vi "FPGA (Top Level)_torque_control.vi"() -> ()   [LabVIEW 2015]
uses:
  <vilib>/Platform/TimedLoop/XDataNode/wakeup.ctl
  <vilib>/Platform/TimedLoop/XDataNode/XDNodeRunTimeDep.lvlib
  <vilib>/Platform/TimedLoop/XDataNode/nitl_modes.ctl
  <vilib>/Platform/TimedLoop/XDataNode/timing_clust.ctl
  <vilib>/Platform/TimedLoop/XDataNode/XDataNode.xnode
  <vilib>/eio/EIONode/EIONode.xnode
  <vilib>/rvi/eio/common/nirviEmuTemplateMethod_errors.vi
  <vilib>/rvi/DataTransferAndStorage/Container/XNode/niFpgaContainer.xnode
  <vilib>/rvi/DataTransferAndStorage/Register/Emulation/niFpgaRegisterEmulation.vi
  <vilib>/rvi/FXPMathLib/FxpSinAndCos/XNode/nifxpmath_SinAndCos.xnode
  <vilib>/rvi/FXPMathLib/FxpSinAndCos/simVIs/DllFxpSinAndCosTemp_sub.vi
  <vilib>/rvi/FXPMathLib/FxpSinAndCos/subVIs/nifxpmath_SinAndCos_SimConfig.ctl
  <vilib>/eio/EIOMethodNode/EIOMethodNode.xnode
  <vilib>/eio/EIOPropertyNode/EIOPropertyNode.xnode
  <vilib>/rvi/eio/common/nirviEmuTemplatePropertyGet_errors.vi
  <vilib>/rvi/eio/common/nirviEmuTemplatePropertyGet_noerrors.vi
  <vilib>/rvi/eio/common/nirviEmuTemplatePropertySet_errors.vi
  <vilib>/rvi/eio/common/nirviEmuTemplatePropertySet_noerrors.vi
  <vilib>/Motion/MotorControl/_s/nism.pwm.v.dcp.range.fxp.1.15.ctl
  <vilib>/rvi/Analysis/control/PID/SubVIs/niFpgaPID_PIWrapper.vi
  <vilib>/Motion/MotorControl/_s/nism.pwm.center.fxp.vi
  <vilib>/LabVIEW Targets/FPGA/cRIO/cRIO-9505/controls.llb/_nicrio_cRIO-9505_DriveStatus.ctl
  <vilib>/rvi/Analysis/control/PID/Typedef/niFpgaPID_PIGains.ctl
  <vilib>/rvi/Analysis/control/PID/Typedef/niFpgaPID_OutputRange.ctl
panel:
  in  "LINK2_DEMAND_CURRENT":sgl
  out "LINK2_ACTUAL_CURRENT":sgl
  in  "LINK2_PI_GAINS":T1 {"proportional gain" step=0.125}
  in  "LINK2_PI_RANGE":T2={"output high (Inf)"=1.0, "output low (-Inf)"=-1.0}
  in  "LINK1_PI_RANGE":T2={"output high (Inf)"=1.0, "output low (-Inf)"=-1.0}
  in  "LINK1_PI_GAINS":T1 {"proportional gain" step=0.125}
  in  "PWM_FREQ":fxp<+,32,0>
  in  "LINK1_DEMAND_CURRENT":sgl
  out "LINK1_ACTUAL_CURRENT":sgl
  out "LINK2_DRIVE_STATUS":T3
  out "LINK1_DRIVE_STATUS":T3
  in  "LINK2_DRIVE_ENABLED":bool
  in  "LINK1_DRIVE_ENABLED":bool
  in  "LINK2_PID_ENABLED":bool
  in  "LINK1_PID_ENABLED":bool
  in  "LINK2_DEMAND_CURRENT":i16
  in  "LINK1_DEMAND_CURRENT":i16
  out "LINK2_ACTUAL_CURRENT":i16
  out "LINK1_ACTUAL_CURRENT":i16
  out "LINK2_X_MM":fxp<+/-,34,16>
  out "LINK2_Y_MM":fxp<+/-,34,16>
  in  "Y_OFFSET_MM":fxp<+/-,33,15>
  in  "X_OFFSET_MM":fxp<+/-,33,15>
  in  "LINK2_LENGTH_MM":fxp<+,16,12>=2.0 format="%#_19g"
  in  "LINK1_LENGTH_MM":fxp<+,16,12>=2.0 format="%#_19g"
  out "LINK2_POT_POS":i32
  out "LINK1_POT_POS":i32
  out "LINK2_ENC_POS":i32
  out "LINK1_ENC_POS":i32
  in  "LINK2_ENC_SCALE":fxp<+,32,0>=0.029296900611370802 format="%#_32g"
  in  "LINK1_ENC_SCALE":fxp<+,32,0> format="%#_32g"
  in  "LINK2_POT_SCALE":fxp<+/-,32,16>
  in  "LINK2_OFFSET":fxp<+/-,16,16>
  in  "LINK1_OFFSET":fxp<+/-,16,16>
  in  "LINK1_POT_SCALE":fxp<+/-,32,16>
  in  "AI_POT_LOOP_US":u16
  in  "ENC_DEBOUNCE_CYCLES":u16=5
  in  "LINK1_ENC_CNTS":i32
  in  "LINK2_ENC_CNTS":i32
  in  "LINK1_UPDATE_ENC":bool
  in  "LINK2_UPDATE_ENC":bool
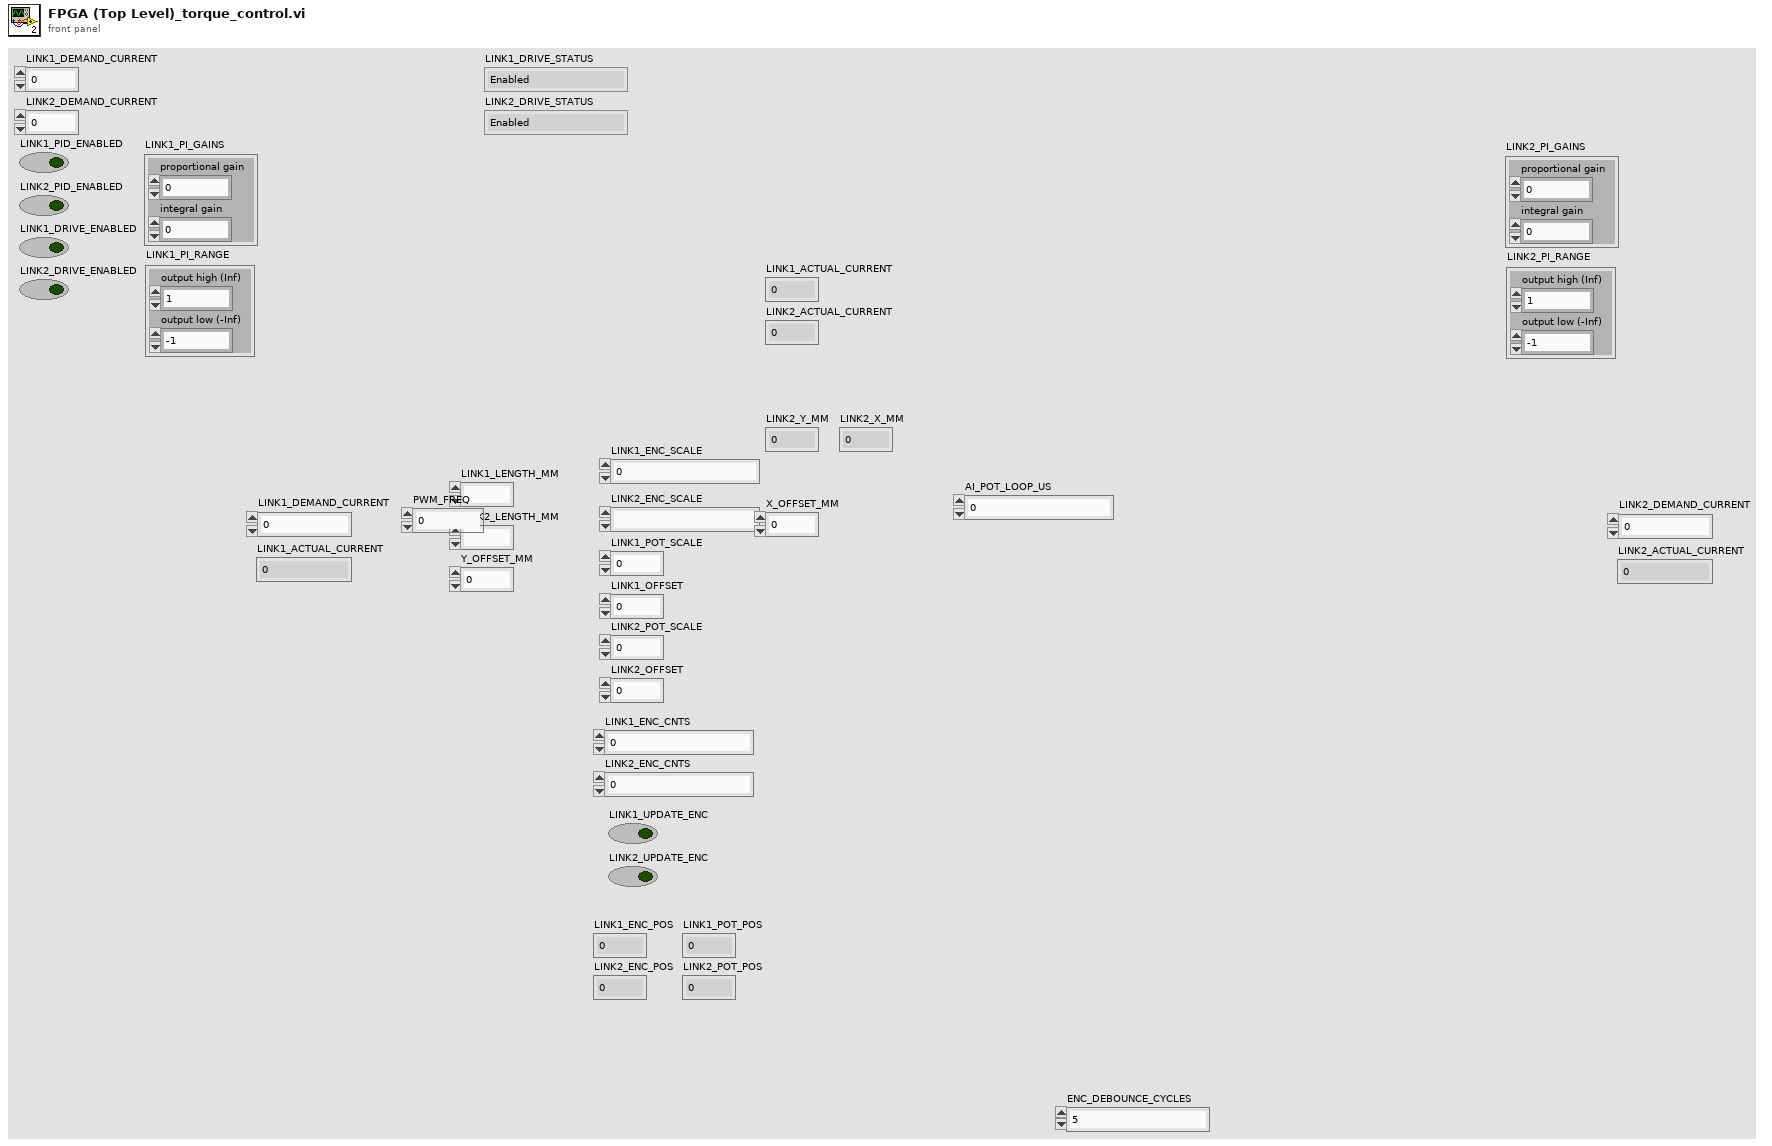
[diagram p1: front panel]
types:
  T1 = typedef "niFpgaPID_PIGains.ctl" = cluster{"proportional gain":sgl, "integral gain":sgl}
  T2 = typedef "niFpgaPID_OutputRange.ctl" = cluster{"output high (Inf)":sgl, "output low (-Inf)":sgl}
  T3 = typedef "_nicrio_cRIO-9505_DriveStatus.ctl" = enum8{"Enabled", "Disabled", "Disabled by Drive Fault", "Disabled by Temp. Fault", "Disabled by E-Stop", "Unknown"}
  T4 = typedef "XDNodeRunTimeDep.lvlib/timing_clust.ctl" = cluster{"Expected End [f-1]":u64, "Actual End [f-1]":u64, "Finished Late? [f-1]":bool, "Expected End [i-1]":u64, "Actual End [i-1]":u64, "Finished Late? [i-1]":bool, "Expected Start [i]":u64, "Actual Start [i]":u64, "Expected Start [f]":u64, "Actual Start [f]":u64, "Source Name":string, "Structure Name":string, "Period":i64, "Deadline":i64, "Offset":i64, "Start":i64, "Priority":i32, "Timeout":i32, "Mode":T5, "Wakeup Reason":T6, "Error":errorcluster, "Source Type":string, "Secondary Source Type":string, "Global End Time":u64, "Global Start Time":u64, "Frame Duration":u64, "Iteration Duration":u64, "Assigned CPU":i32, "I/O Scan Engine Mode":u32}
  T5 = typedef "XDNodeRunTimeDep.lvlib/nitl_modes.ctl" = enum32{"No Change", "Process missed periods, maintain original phase", "Discard missed periods, maintain original phase", "Process missed periods, ignore original phase", "Discard missed periods, ignore original phase"}
  T6 = typedef "XDNodeRunTimeDep.lvlib/wakeup.ctl" = enum32{"Normal", "Aborted", "Asynchronous wakeup", "Timing source error", "Timed loop error", "Timeout"}
  T7 = typedef "NI_SoftMotion_MotorControlIP.lvlib/nism.pwm.v.dcp.range.fxp.1.15.ctl" = cluster{"upper limit":fxp<+,16,1>, "lower limit":fxp<+,16,1>}
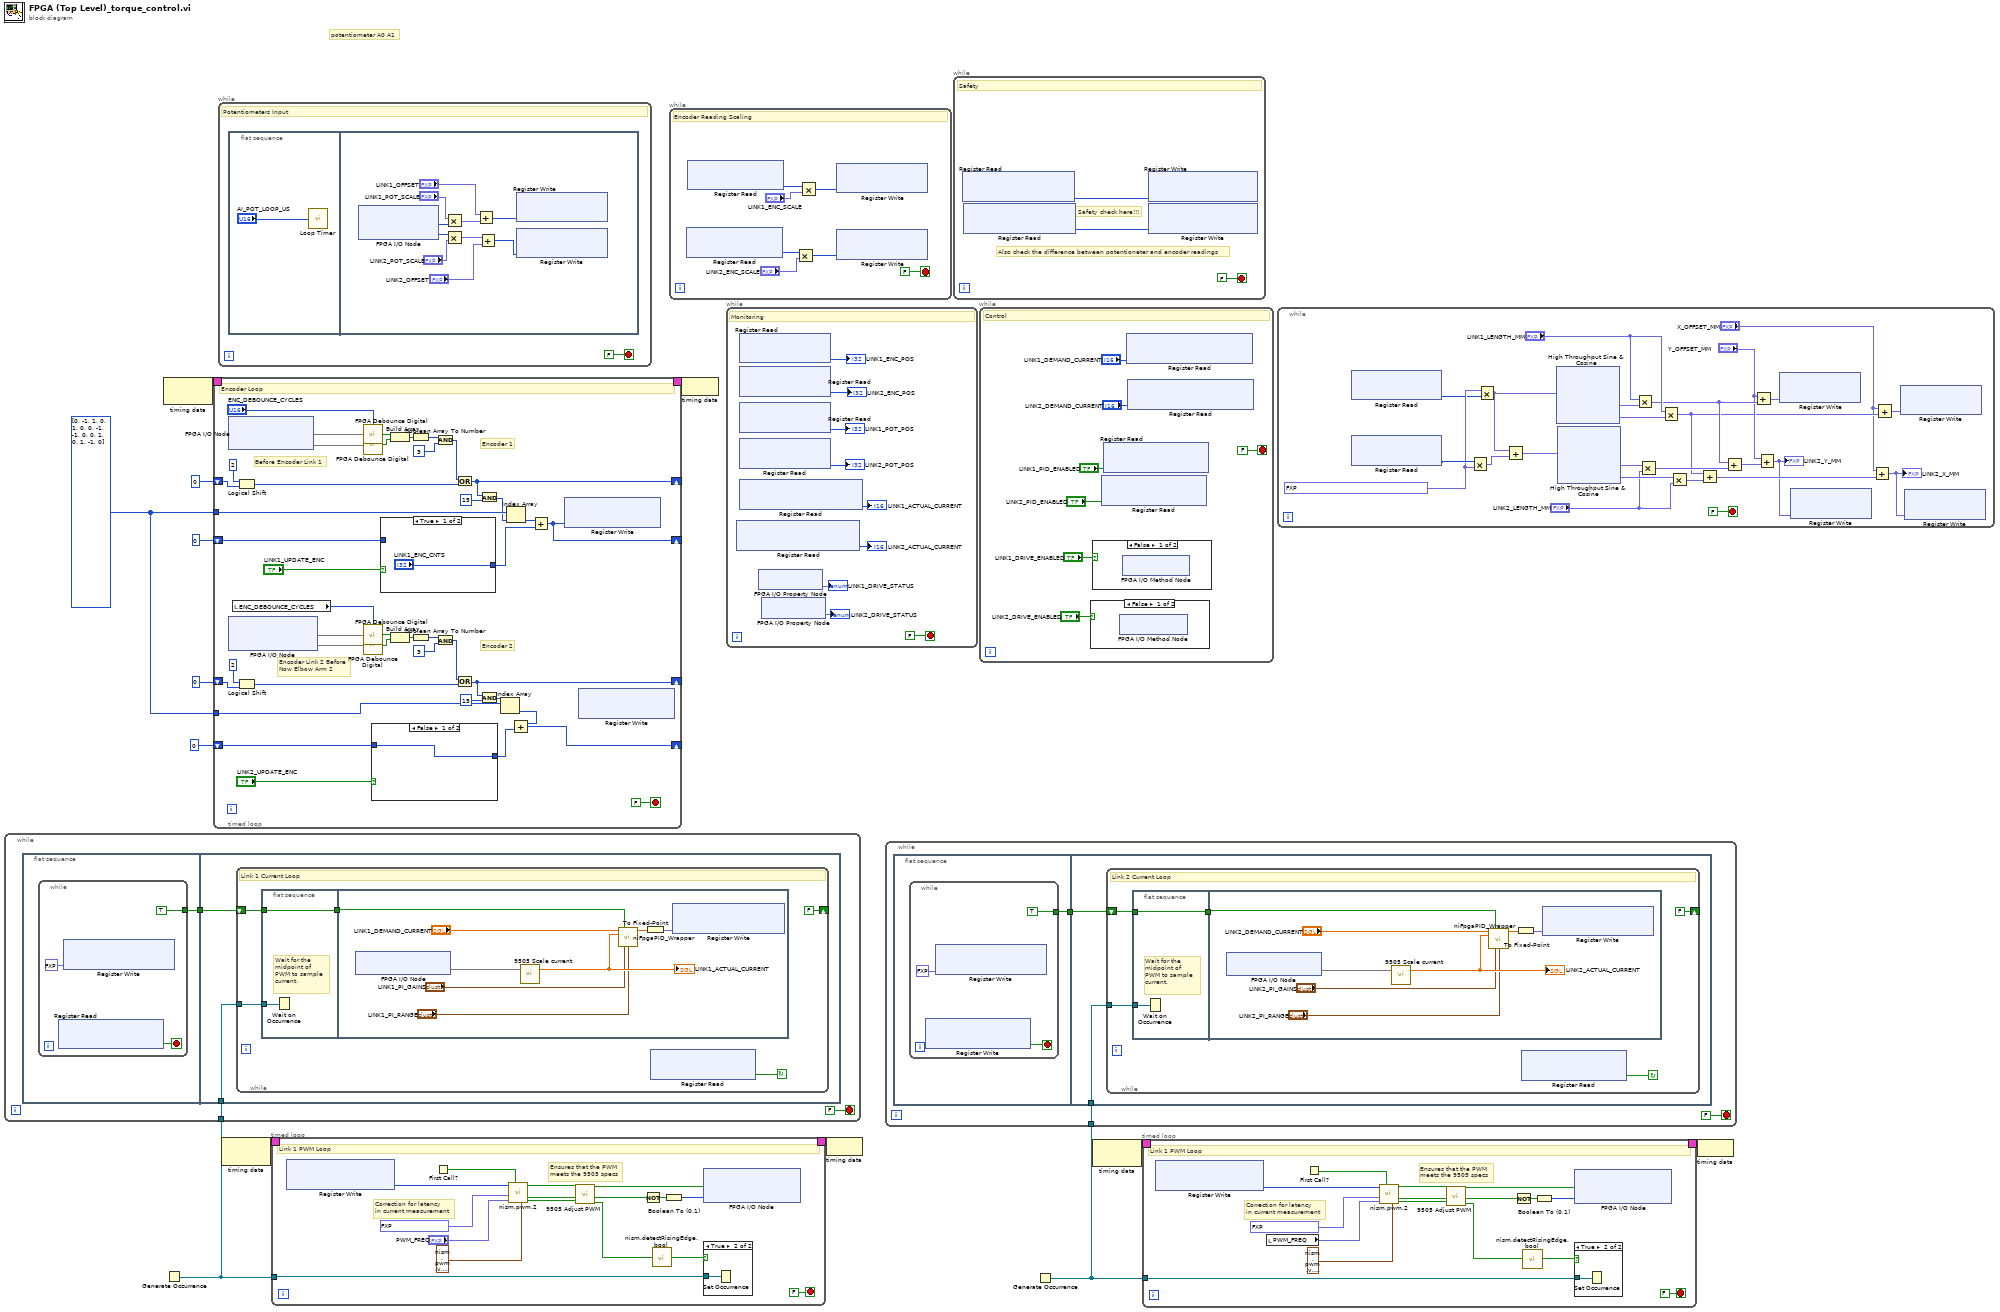
[diagram p0: block diagram]
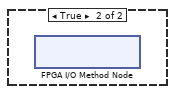
[diagram p4: hidden frame]
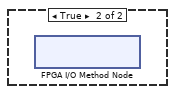
[diagram p5: hidden frame]
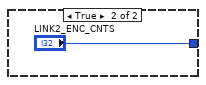
[diagram p6: hidden frame]
diagram:
  w9 = i8[] [0, -1, 1, 0, 1, 0, 0, -1, -1, 0, 0, 1, 0, 1, -1, 0]
  # "potentiometer A0 A1"
  n1 = node-c288() -> (w13:T4)  [unwired: 1 in]
  n2 = Generate Occurrence ("Current\nSample\nSync")() -> (w4:refnum<k4>)
  n3 = while {
    tunnel: w4 -> [w15]
    stop <- FALSE stop-if-true
    n4 = flat-sequence {
      tunnel: [w17] -> w16
      tunnel: w15 -> [w22]
      tunnel: w16 -> [w21]
      frame #0 {
        n5 = while {
          tunnel: [TRUE] -> w17
          stop <- w19 stop-if-true
          n6 = xnode ("Register Read")() -> ("Data"=w19:bool)  [unwired: 1 in, 1 out]
          n7 = xnode "Register Write"("Data"=fxp<+/-,16,1> 0.0) -> ()  [unwired: 1 in, 1 out]
        }
      }
      frame #1 {
        n8 = while "FOC and Halls" {
          tunnel: w22 -> [w27]
          shift-right: [FALSE] -> _
          shift-left: w21 -> [w25]
          stop <- w23 continue-if-true
          # "Link 1 Current Loop"
          n9 = flat-sequence {
            tunnel: w27 -> [w29]
            tunnel: [w28] -> w26
            tunnel: w25 -> [w28]
            tunnel: w26 -> [w31]
            frame #0 {
              # "Wait for the \nmidpoint of \nPWM to sample \ncurrent."
              n10 = Wait on Occurrence(2:w29) -> ()  [unwired: 2 in, 1 out]
            }
            frame #1 {
              n11 = xnode "FPGA I/O Node"() -> ("Link 1/Current Sense"=w36)  [unwired: 1 in, 1 out]
              n12 = call "9505 Scale current.vi"("Current Reading"=w36) -> ("Actual Current (Amps)"=w35:sgl)  [unwired: 18 in]
              "LINK1_ACTUAL_CURRENT" <- w35
              n13 = call-poly <vilib>:"niFpgaPID_Wrapper.vi"("setpoint"="LINK1_DEMAND_CURRENT", "reset? (F)"=w31, "process variable"=w35, "gains"="LINK1_PI_GAINS", "output range"="LINK1_PI_RANGE") -> ("output"=w37:sgl)  [unwired: 8 in, 2 out]
              n14 = To Fixed-Point(number=w37) -> (fixed-point=w32:fxp<+/-,16,1>)  [unwired: 1 in]
              n15 = xnode "Register Write"("Data"=w32) -> ()  [unwired: 1 in, 1 out]
            }
          }
          n16 = xnode ("Register Read")() -> ("Data"=w23:bool)  [unwired: 1 in, 1 out]
        }
      }
    }
  }
  n17 = timed-loop {
    timing: w13 -> [_]
    timing-out: [_] -> w12
    tunnel: w9 -> [w77]
    shift-right: [w70] -> _
    shift-left: u8 0 -> [w79]
    shift-right: [w41] -> _
    shift-left: 0 -> [w62]
    tunnel: w9 -> [w46]
    shift-right: [w44] -> _
    shift-left: u8 0 -> [w45]
    shift-right: [w40] -> _
    shift-left: 0 -> [w38]
    stop <- FALSE stop-if-true
    # "Encoder Link 2 Before\nNow Elbow Arm 2"
    # "Before Encoder Link 1"
    # "Encoder 2"
    # "Encoder 1"
    # "Encoder Loop"
    n18 = xnode "FPGA I/O Node"() -> ("ConnectorA/DIO8"=w68, "ConnectorA/DIO9"=w67)  [unwired: 2 in, 2 out]
    n19 = xnode "FPGA I/O Node"() -> ("ConnectorA/DIO10"=w52, "ConnectorA/DIO11"=w51)  [unwired: 2 in, 2 out]
    n20 = local read "ENC_DEBOUNCE_CYCLES"() -> (w43:u16)
    n21 = Logical Shift(y=i16 2, x=w79) -> (x << y=w72:u8)
    n22 = Logical Shift(y=i16 2, x=w45) -> (x << y=w55:u8)
    n23 = call "FPGA Debounce Digital.vi"("Input Signal"=w68, "Cycles to Filter"="ENC_DEBOUNCE_CYCLES") -> ("Output Filtered Signal"=w66:bool)
    n24 = call "FPGA Debounce Digital.vi"("Input Signal"=w67, "Cycles to Filter"="ENC_DEBOUNCE_CYCLES") -> ("Output Filtered Signal"=w65:bool)
    n25 = call "FPGA Debounce Digital.vi"("Input Signal"=w52, "Cycles to Filter"=w43) -> ("Output Filtered Signal"=w50:bool)
    n26 = call "FPGA Debounce Digital.vi"("Input Signal"=w51, "Cycles to Filter"=w43) -> ("Output Filtered Signal"=w49:bool)
    n27 = case shown="False" "LINK2_UPDATE_ENC" {
      tunnel: w38 -> [w81 _]
      tunnel: [w81 "LINK2_ENC_CNTS"] -> w47
      frame False {
      }
      frame True {
      }
    }
    n28 = case shown="True" "LINK1_UPDATE_ENC" {
      tunnel: w62 -> [_ w84]
      tunnel: ["LINK1_ENC_CNTS" w84] -> w61
      frame True {
      }
      frame False {
      }
    }
    n29 = Build Array(w66, w65) -> (w64:bool[])
    n30 = Build Array(w50, w49) -> (w48:bool[])
    n31 = Boolean Array To Number(Boolean array=w64) -> (number=w75:u8)
    n32 = Boolean Array To Number(Boolean array=w48) -> (number=w58:u8)
    n33 = And(x=w75, y=u8 3) -> (x .and. y?=w73:u8)
    n34 = And(x=w58, y=u8 3) -> (x .and. y?=w56:u8)
    n35 = Or(x=w73, y=w72) -> (x .or. y?=w70:u8)
    n36 = Or(x=w56, y=w55) -> (x .or. y?=w44:u8)
    n37 = And(x=w70, y=u8 15) -> (x .and. y?=w71:u8)
    n38 = And(x=w44, y=u8 15) -> (x .and. y?=w54:u8)
    n39 = Index Array(array=w46, index=w54) -> (element=w53:i8)
    n40 = Index Array(array=w77, index=w71) -> (element=w69:i8)
    n41 = Add(x=w53, y=w47) -> (x+y=w40:i32)
    n42 = Add(x=w69, y=w61) -> (x+y=w41:i32)
    n43 = xnode ("Register Write")("Data"=w41) -> ()  [unwired: 1 in, 1 out]
    n44 = xnode ("Register Write")() -> ()  [unwired: 2 in, 1 out]
  }
  n45 = while {
    stop <- FALSE stop-if-true
    # "Potentiometers Input"
    n46 = flat-sequence {
      frame #0 {
        n47 = call "Loop Timer"("Count(uSec)"="AI_POT_LOOP_US") -> ()  [unwired: 1 out]
      }
      frame #1 {
        n48 = xnode "FPGA I/O Node"() -> ("ConnectorA/AI0"=w98:u16, "ConnectorA/AI1"=w92:u16)  [unwired: 2 in, 2 out]
        n49 = Multiply(x="LINK1_POT_SCALE", y=w98) -> (x*y=w96:fxp<+/-,48,32>)
        n50 = Multiply(x=w92, y="LINK2_POT_SCALE") -> (x*y=w91:fxp<+/-,48,32>)
        n51 = Add(x="LINK1_OFFSET", y=w96) -> (x+y=w90:i32)
        n52 = Add(x=w91, y="LINK2_OFFSET") -> (x+y=w89:i32)
        n53 = xnode ("Register Write")("Data"=w90) -> ()  [unwired: 1 in, 1 out]
        n54 = xnode ("Register Write")("Data"=w89) -> ()  [unwired: 1 in, 1 out]
      }
    }
  }
  n55 = node-c288() -> (w6:T4)  [unwired: 1 in]
  n56 = timed-loop "PWM Generation" {
    timing: w6 -> [_]
    timing-out: [_] -> w5
    tunnel: w4 -> [w114]
    stop <- FALSE stop-if-true
    # "Correction for latency\nin current measurement"
    # "Ensures that the PWM\nmeets the 9505 specs"
    # "Link 1 PWM Loop"
    n57 = xnode "Register Write"() -> ("Data"=w99:i16)  [unwired: 1 in, 1 out]
    n58 = First Call?() -> (First Call?: T/F=w111:bool)
    n59 = call-poly <vilib>:"nism.pwm.2.vi"("range"=T7 {"upper limit"=1.0, "lower limit"=0.0} ("PWM Range"), "reset"=w111, "frequency"="PWM_FREQ", "trigger lead"=fxp<+/-,16,1> -0.004913330078125, "duty cycle"=w99) -> ("direction"=w103:bool, "trigger"=w102:bool, "pwm"=w101:bool)  [unwired: 4 in]
    n60 = call "9505 Adjust PWM.vi"("Direction"=w103, "Trigger"=w102, "PWM"=w101) -> ("Trigger Out"=w106:bool, "Direction Out"=w104:bool, "Output PWM"=w105:bool)  [unwired: 6 in]
    n61 = Not(x=w104) -> (.not. x?=w108:bool)
    n62 = call <vilib>:"nism.detectRisingEdge.bool.vi"("x"=w106) -> ("y"=w110:bool)
    n63 = Boolean To (0,1)(Boolean=w108) -> (0, 1=w109:i16)
    n64 = xnode "FPGA I/O Node"("Link 1/Motor"=w105, "Link 1/Drive Direction"=w109) -> ()  [unwired: 2 in, 2 out]
    n65 = case shown="True" w110 {
      tunnel: w114 -> [_ w115]
      frame False {
      }
      frame True {
        n66 = Set Occurrence(w115) -> ()
      }
    }
  }
  n67 = while {
    stop <- FALSE stop-if-true
    # "Encoder Reading Scaling"
    n68 = xnode ("Register Read")() -> ("Data"=w123:i32)  [unwired: 1 in, 1 out]
    n69 = xnode ("Register Read")() -> ("Data"=w121:i32)  [unwired: 1 in, 1 out]
    n70 = Multiply(x=w123, y="LINK2_ENC_SCALE") -> (x*y=w118:i32)
    n71 = Multiply(x=w121, y="LINK1_ENC_SCALE") -> (x*y=w120:i32)
    n72 = xnode ("Register Write")("Data"=w120) -> ()  [unwired: 1 in, 1 out]
    n73 = xnode ("Register Write")("Data"=w118) -> ()  [unwired: 1 in, 1 out]
  }
  n74 = node-c288(w12) -> ()
  n75 = while {
    stop <- FALSE stop-if-true
    # "Monitoring"
    n76 = xnode ("Register Read")() -> ("Data"=→"LINK2_ACTUAL_CURRENT":i16)  [unwired: 1 in, 1 out]
    n77 = xnode ("Register Read")() -> ("Data"=→"LINK1_ENC_POS":i32)  [unwired: 1 in, 1 out]
    n78 = xnode ("Register Read")() -> ("Data"=→"LINK2_ENC_POS":i32)  [unwired: 1 in, 1 out]
    n79 = xnode ("Register Read")() -> ("Data"=→"LINK1_POT_POS":i32)  [unwired: 1 in, 1 out]
    n80 = xnode ("Register Read")() -> ("Data"=→"LINK2_POT_POS":i16)  [unwired: 1 in, 1 out]
    n81 = xnode ("Register Read")() -> ("Data"=→"LINK1_ACTUAL_CURRENT":i16)  [unwired: 1 in, 1 out]
    n82 = xnode "FPGA I/O Property Node"() -> ("Drive Status"=→"LINK1_DRIVE_STATUS")  [unwired: 1 in, 1 out]
    n83 = xnode "FPGA I/O Property Node"() -> ("Drive Status"=→"LINK2_DRIVE_STATUS")  [unwired: 1 in, 1 out]
  }
  n84 = node-c288(w5) -> ()
  n85 = while {
    stop <- FALSE stop-if-true
    # "Also check the difference between potentioneter and encoder readings"
    # "Do Safety check here!!!"
    # "Safety"
    n86 = xnode ("Register Read")() -> ("Data"=w135:i16)  [unwired: 1 in, 1 out]
    n87 = xnode ("Register Read")() -> ("Data"=w134:i16)  [unwired: 1 in, 1 out]
    n88 = xnode ("Register Write")("Data"=w135) -> ()  [unwired: 1 in, 1 out]
    n89 = xnode ("Register Write")("Data"=w134) -> ()  [unwired: 1 in, 1 out]
  }
  n90 = while {
    stop <- FALSE stop-if-true
    # "Control"
    n91 = case shown="False" "LINK2_DRIVE_ENABLED" {
      frame False {
        n92 = xnode "FPGA I/O Method Node"() -> ()  [unwired: 1 in, 1 out]
      }
      frame True {
        n93 = xnode "FPGA I/O Method Node"() -> ()  [unwired: 1 in, 1 out]
      }
    }
    n94 = case shown="False" "LINK1_DRIVE_ENABLED" {
      frame False {
        n95 = xnode "FPGA I/O Method Node"() -> ()  [unwired: 1 in, 1 out]
      }
      frame True {
        n96 = xnode "FPGA I/O Method Node"() -> ()  [unwired: 1 in, 1 out]
      }
    }
    n97 = xnode ("Register Read")("Data"="LINK2_PID_ENABLED") -> ()  [unwired: 1 in, 1 out]
    n98 = xnode ("Register Read")("Data"="LINK1_PID_ENABLED") -> ()  [unwired: 1 in, 1 out]
    n99 = xnode ("Register Read")("Data"="LINK1_DEMAND_CURRENT") -> ()  [unwired: 1 in, 1 out]
    n100 = xnode ("Register Read")("Data"="LINK2_DEMAND_CURRENT") -> ()  [unwired: 1 in, 1 out]
  }
  n101 = Generate Occurrence ("Current\nSample\nSync")() -> (w1:refnum<k4>)
  n102 = while {
    tunnel: w1 -> [w145]
    stop <- FALSE stop-if-true
    n103 = flat-sequence {
      tunnel: [w147] -> w146
      tunnel: w145 -> [w152]
      tunnel: w146 -> [w151]
      frame #0 {
        n104 = while {
          tunnel: [TRUE] -> w147
          stop <- w148 stop-if-true
          n105 = xnode "Register Write"() -> ("Data"=w148:bool)  [unwired: 1 in, 1 out]
          n106 = xnode "Register Write"("Data"=fxp<+/-,16,1> 0.0) -> ()  [unwired: 1 in, 1 out]
        }
      }
      frame #1 {
        n107 = while "FOC and Halls" {
          tunnel: w152 -> [w157]
          shift-right: [FALSE] -> _
          shift-left: w151 -> [w155]
          stop <- w153 continue-if-true
          # "Link 2 Current Loop"
          n108 = flat-sequence {
            tunnel: w157 -> [w159]
            tunnel: [w158] -> w156
            tunnel: w155 -> [w158]
            tunnel: w156 -> [w162]
            frame #0 {
              # "Wait for the \nmidpoint of \nPWM to sample \ncurrent."
              n109 = Wait on Occurrence(2:w159) -> ()  [unwired: 2 in, 1 out]
            }
            frame #1 {
              n110 = xnode "FPGA I/O Node"() -> ("Link 2/Current Sense"=w166)  [unwired: 1 in, 1 out]
              n111 = call "9505 Scale current.vi"("Current Reading"=w166) -> ("Actual Current (Amps)"=w165:sgl)  [unwired: 18 in]
              "LINK2_ACTUAL_CURRENT" <- w165
              n112 = call-poly <vilib>:"niFpgaPID_Wrapper.vi"("setpoint"="LINK2_DEMAND_CURRENT", "reset? (F)"=w162, "process variable"=w165, "gains"="LINK2_PI_GAINS", "output range"="LINK2_PI_RANGE") -> ("output"=w167:sgl)  [unwired: 8 in, 2 out]
              n113 = To Fixed-Point(number=w167) -> (fixed-point=w160:fxp<+/-,16,1>)  [unwired: 1 in]
              n114 = xnode "Register Write"("Data"=w160) -> ()  [unwired: 1 in, 1 out]
            }
          }
          n115 = xnode ("Register Read")() -> ("Data"=w153:bool)  [unwired: 1 in, 1 out]
        }
      }
    }
  }
  n116 = node-c288() -> (w3:T4)  [unwired: 1 in]
  n117 = timed-loop "PWM Generation" {
    timing: w3 -> [_]
    timing-out: [_] -> w2
    tunnel: w1 -> [w183]
    stop <- FALSE stop-if-true
    # "Correction for latency\nin current measurement"
    # "Ensures that the PWM\nmeets the 9505 specs"
    # "Link 1 PWM Loop"
    n118 = xnode "Register Write"() -> ("Data"=w169:i16)  [unwired: 1 in, 1 out]
    n119 = local read "PWM_FREQ"() -> (w168:fxp<+,32,0>)
    n120 = First Call?() -> (First Call?: T/F=w181:bool)
    n121 = call-poly <vilib>:"nism.pwm.2.vi"("range"=T7 {"upper limit"=1.0, "lower limit"=0.0} ("PWM Range"), "reset"=w181, "frequency"=w168, "trigger lead"=fxp<+/-,16,1> -0.004913330078125, "duty cycle"=w169) -> ("direction"=w173:bool, "trigger"=w172:bool, "pwm"=w171:bool)  [unwired: 4 in]
    n122 = call "9505 Adjust PWM.vi"("Direction"=w173, "Trigger"=w172, "PWM"=w171) -> ("Trigger Out"=w176:bool, "Direction Out"=w174:bool, "Output PWM"=w175:bool)  [unwired: 6 in]
    n123 = Not(x=w174) -> (.not. x?=w178:bool)
    n124 = call <vilib>:"nism.detectRisingEdge.bool.vi"("x"=w176) -> ("y"=w180:bool)
    n125 = Boolean To (0,1)(Boolean=w178) -> (0, 1=w179:i16)
    n126 = xnode "FPGA I/O Node"("Link 2/Motor"=w175, "Link 2/Drive Direction"=w179) -> ()  [unwired: 2 in, 2 out]
    n127 = case shown="True" w180 {
      tunnel: w183 -> [_ w184]
      frame False {
      }
      frame True {
        n128 = Set Occurrence(w184) -> ()
      }
    }
  }
  n129 = while {
    stop <- FALSE stop-if-true
    w193 = fxp<+,31,-8> 5.555555617320351e-05
    n130 = xnode ("Register Read")() -> ("Data"=w192:i32)  [unwired: 1 in, 1 out]
    n131 = xnode ("Register Read")() -> ("Data"=w210:i32)  [unwired: 1 in, 1 out]
    n132 = Multiply(x=w210, y=w193) -> (x*y=w209:fxp<+/-,63,24>)
    n133 = Multiply(x=w193, y=w192) -> (x*y=w191:fxp<+/-,63,24>)
    n134 = Add(x=w191, y=w209) -> (x+y=w208:fxp<+/-,64,25>)
    n135 = xnode "High Throughput Sine & Cosine"("x (pi)"=w191) -> ("sin(x)"=w207:fxp<+/-,16,2>, "cos(x)"=w206:fxp<+/-,16,2>)
    n136 = xnode "High Throughput Sine & Cosine"("x (pi)"=w208) -> ("sin(x)"=w204:fxp<+/-,16,2>, "cos(x)"=w203:fxp<+/-,16,2>)
    n137 = Multiply(x="LINK1_LENGTH_MM", y=w207) -> (x*y=w199:fxp<+/-,32,14>)
    n138 = Multiply(x=w204, y="LINK2_LENGTH_MM") -> (x*y=w200:fxp<+/-,32,14>)
    n139 = Multiply(x="LINK1_LENGTH_MM", y=w206) -> (x*y=w196:fxp<+/-,32,14>)
    n140 = Multiply(x=w203, y="LINK2_LENGTH_MM") -> (x*y=w201:fxp<+/-,32,14>)
    n141 = Add(x=w196, y=w201) -> (x+y=w195:fxp<+/-,33,15>)
    n142 = Add(x=w199, y=w200) -> (x+y=w198:fxp<+/-,33,15>)
    n143 = Add(x="Y_OFFSET_MM", y=w199) -> (x+y=w190:fxp<+/-,34,16>)
    n144 = Add(x="Y_OFFSET_MM", y=w198) -> (x+y=w188:fxp<+/-,34,16>)
    "LINK2_Y_MM" <- w188
    n145 = xnode ("Register Write")("Data"=w190) -> ()  [unwired: 1 in, 1 out]
    n146 = xnode ("Register Write")("Data"=w188) -> ()  [unwired: 1 in, 1 out]
    n147 = Add(x="X_OFFSET_MM", y=w195) -> (x+y=w187:fxp<+/-,34,16>)
    "LINK2_X_MM" <- w187
    n148 = Add(x="X_OFFSET_MM", y=w196) -> (x+y=w189:fxp<+/-,34,16>)
    n149 = xnode ("Register Write")("Data"=w189) -> ()  [unwired: 1 in, 1 out]
    n150 = xnode ("Register Write")("Data"=w187) -> ()  [unwired: 1 in, 1 out]
  }
  n151 = node-c288(w2) -> ()
